vi "Write Pulse Mode.vi"(8 "error in":errorcluster, 10 "Pulse Mode":T1, 11 "3300 in":refnum<class "3300.lvclass">) -> (0 "error out":errorcluster, 3 "3300 out":refnum<class "3300.lvclass">)   [LabVIEW 2019, in "3300.lvlib" / "3300.lvclass"]
uses:
  Library/3300.lvclass
  builds/Instruments/Electronic Load.lvlibp/Custom Controls/E-Load Mode.ctl
  builds/Instruments/Electronic Load.lvlibp/Library/Electronic Load.lvclass
  builds/Engine/Engine.lvlibp/Project/Engine.lvclass
  C:/Users/Public/Documents/Development/builds/Engine/Engine.lvlibp/Project/Engine.lvclass
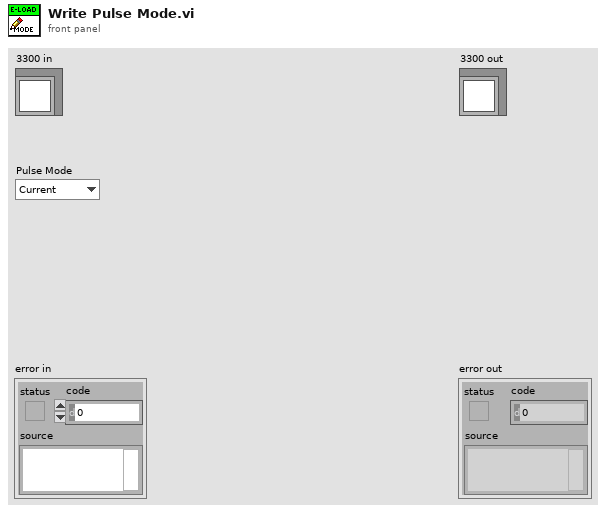
[diagram p1: front panel]
types:
  T1 = typedef "Electronic Load.lvlibp/Electronic Load.lvclass/E-Load Mode.ctl" = enum16{"Current", "Resistance", "Voltage"}
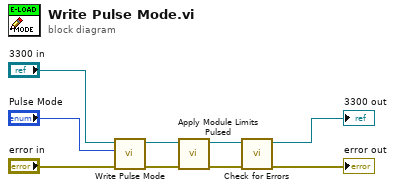
[diagram p0: block diagram]
diagram:
  n1 = call-parent "Write Pulse Mode.vi"("error in"="error in", "Pulse Mode"="Pulse Mode", "Electronic Load in"="3300 in") -> ("error out"=w6:errorcluster, "Electronic Load out"=w5:refnum<class "3300.lvclass">)  [unwired: 7 in]
  n2 = call "Apply Module Limits Pulsed.vi"("error in"=w6, "3300 in"=w5) -> ("error out"=w3:errorcluster, "3300 out"=w4:refnum<class "3300.lvclass">)  [unwired: 8 in]
  n3 = call "Check for Errors.vi"("error in"=w3, "Engine in"=w4) -> ("error out"=→"error out":errorcluster, "Engine out"=→"3300 out":refnum<class "3300.lvclass">)  [unwired: 8 in]
